vi "Write to 2.vi"(11 "Test Case In":refnum<class "Tests Event MessengerM.lvclass">) -> (0 "error out":errorcluster, 3 "Test Case Out":refnum<class "Tests Event MessengerM.lvclass">)   [LabVIEW 2020, in "Tests Event MessengerM.lvclass"]
uses:
  Tests Event MessengerM.lvclass
  C:/Program Files/National Instruments/LabVIEW 2026/vi.lib/Astemes/LUnit/Test Case.lvclass
  <vilib>/Astemes/LUnit/Test Case.lvclass/Test Case.ctl
  <vilib>/Astemes/LUnit/Test Case.lvclass
  96d37a62-d373-4009-9144-224a0ab690da.vi
  2aeb12fe-a986-4636-b63d-54def23091b0.vi
  7db9f443-421b-401e-8f5d-804821fbaef7.vi
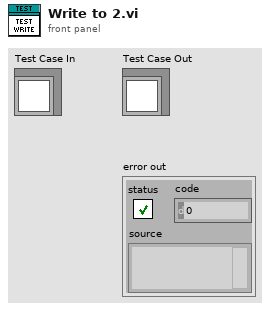
[diagram p1: front panel]
types:
  T1 = typedef "Event MessengerM-c(str,var).lvlib/))Channel.ctl" = refnum<queue>
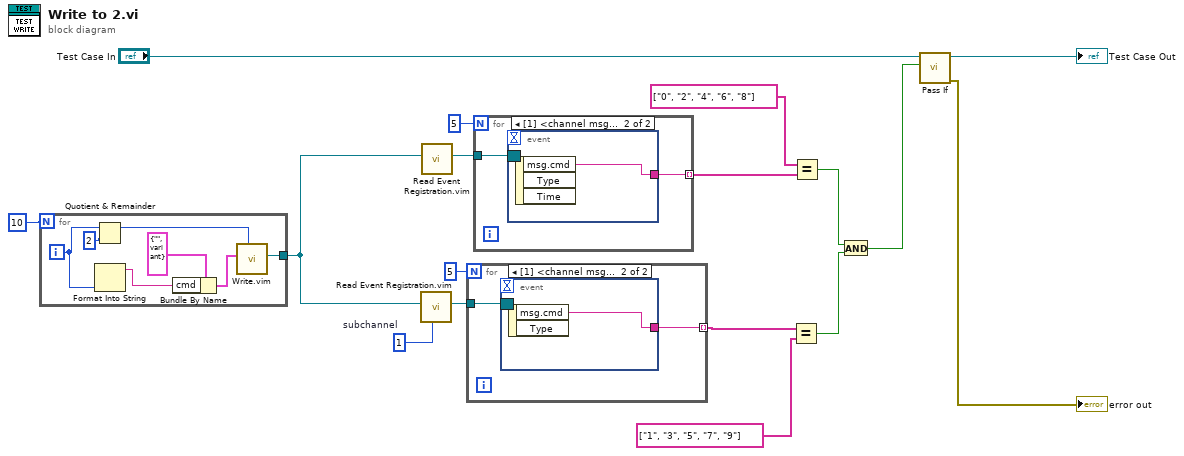
[diagram p0: block diagram]
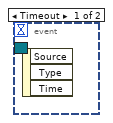
[diagram p2: hidden frame]
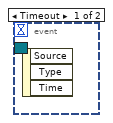
[diagram p3: hidden frame]
diagram:
  w1 = 1  # subchannel
  n1 = for {
    N: 10 -> [_]
    tunnel: [w18] -> w4
    i -> [w22]
    n2 = Quotient & Remainder(x=w22, y=2) -> (x-y*floor(x/y)=w19:i32)  [unwired: 1 out]
    n3 = Format Into String(w22) -> (resulting string=w21:string)  [unwired: 3 in, 1 out]
    n4 = Bundle By Name(cluster=cluster{"cmd":string, "data":variant} {"cmd"="", "data"=variant} ("element"), "cmd"=w21) -> (w20:cluster{"cmd":string, "data":variant})
    n5 = call "Write.vim"("subchannel"=w19, "element"=w20) -> ("channel"=w18:T1)  [unwired: 8 in, 1 out]
  }
  n6 = call "Read Event Registration.vim"("subchannel"=w1, "channel"=w4) -> ("event registration refnum"=w2:refnum<event-registration>)  [unwired: 9 in]
  n7 = call "Read Event Registration.vim"("channel"=w4) -> ("event registration refnum"=w3:refnum<event-registration>)  [unwired: 10 in]
  n8 = for {
    N: 5 -> [_]
    tunnel: w2 -> [w26]
    tunnel: [w25] -> w11 mode=indexing
    n9 = event shown="[1] <channel msg>: User Event" {
      selector: w26 -> [_ _]
      dyn-events: _ -> [_ _]
      timeout: _ -> [_ _]
      tunnel: [_ w27] -> w25
      event Timeout {
        n10 = event-data() -> ()  [unwired: 1 in, 3 out]
      }
      event User Event {
        n11 = event-data() -> ("msg.cmd"=w27:string)  [unwired: 1 in, 1 out]
      }
    }
  }
  n12 = for {
    N: 5 -> [_]
    tunnel: w3 -> [w29]
    tunnel: [w28] -> w8 mode=indexing
    n13 = event shown="[1] <channel msg>: User Event" {
      selector: w29 -> [_ _]
      dyn-events: _ -> [_ _]
      timeout: _ -> [_ _]
      tunnel: [_ w30] -> w28
      event Timeout {
        n14 = event-data() -> ()  [unwired: 1 in, 3 out]
      }
      event User Event {
        n15 = event-data() -> ("msg.cmd"=w30:string)  [unwired: 1 in, 2 out]
      }
    }
  }
  n16 = Equal?(x=w11, y=string[] ["1", "3", "5", "7", "9"] ("Array 2")) -> (x = y?=w9:bool)
  n17 = Equal?(x=string[] ["0", "2", "4", "6", "8"] ("Array"), y=w8) -> (x = y?=w6:bool)
  n18 = And(x=w6, y=w9) -> (x .and. y?=w5:bool)
  n19 = call <vilib>:"Pass If.vi"("Pass?"=w5, "LUnit Test Case In"="Test Case In") -> ("error out"=→"error out":errorcluster, "LUnit Test Case Out"=→"Test Case Out":refnum<class "Tests Event MessengerM.lvclass">)  [unwired: 8 in]
